vi "write comment cell with column offset.vi"(5 "Column Relative?":bool, 6 "comment string":string, 7 "Row offset":i32, 8 "error in (no error)":errorcluster, 9 "comment column offset":i32, 10 "start of last occupied row":cluster{"row":i32, "column":i32}, 11 "NI_report in":refnum<class "NI_report.lvclass">) -> (0 "error out":errorcluster, 3 "NI_report out":refnum<class "NI_report.lvclass">)   [LabVIEW 2016]
uses:
  <vilib>/Utility/NIReport.llb/NI_report.lvclass
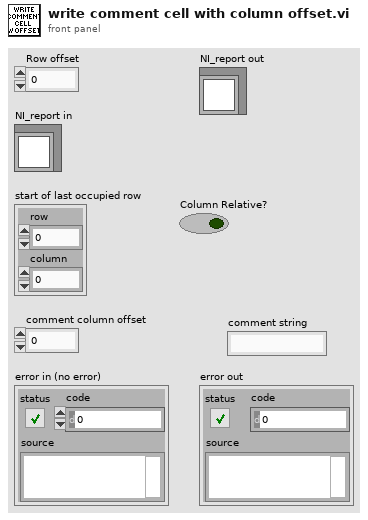
[diagram p1: front panel]
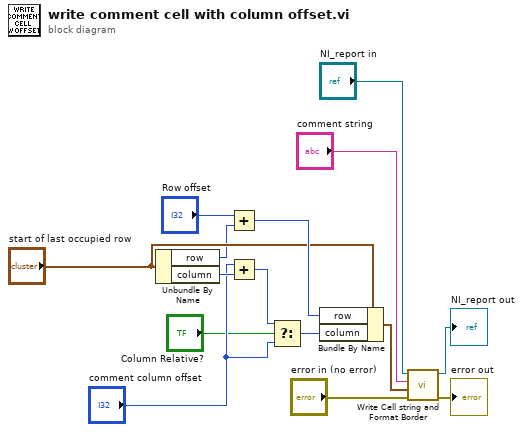
[diagram p0: block diagram]
diagram:
  n1 = Unbundle By Name("start of last occupied row") -> ("row"=w6:i32, "column"=w15:i32)
  n2 = Add(x="Row offset", y=w6) -> (x+y=w9:i32)
  n3 = Add(x="comment column offset", y=w15) -> (x+y=w3:i32)
  n4 = Select(t=w3, s="Column Relative?", f="comment column offset") -> (s? t:f=w4:i32)
  n5 = Bundle By Name(cluster="start of last occupied row", "row"=w9, "column"=w4) -> (w11:cluster{"row":i32, "column":i32})
  n6 = call "Write Cell string and Format Border.vi"("error in (no error)"="error in (no error)", "output cluster"=w11, "input string"="comment string", "NI_report in"="NI_report in") -> ("error out"=→"error out":errorcluster, "NI_report out"=→"NI_report out":refnum<class "NI_report.lvclass">)  [unwired: 6 in]
